vi "Time difference.vi"(10 "Start time":timestamp, 11 "Current time":timestamp) -> (3 "Difference (sec)":i64)   [LabVIEW 2015]
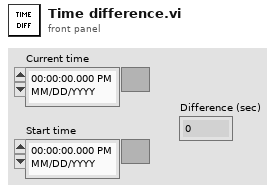
[diagram p1: front panel]
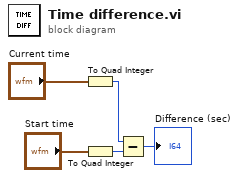
[diagram p0: block diagram]
diagram:
  n1 = To Quad Integer(1:"Current time") -> (0:w4:i64)
  n2 = To Quad Integer(1:"Start time") -> (0:w5:i64)
  n3 = Subtract(x=w4, y=w5) -> (x-y=→"Difference (sec)":i64)
